vi "WPI_ERRMotorControlCANJaguarFirmware.vi"(0 "error code":i32, 7 "Device Number":u8, 9 "minimum firmware version":u32, 11 "current firmware version":u32) -> (8 "error out":errorcluster)   [LabVIEW 2017]
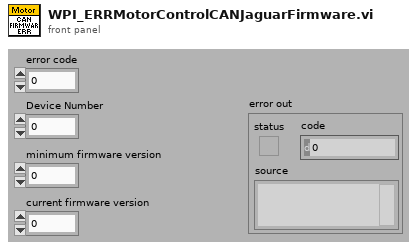
[diagram p1: front panel]
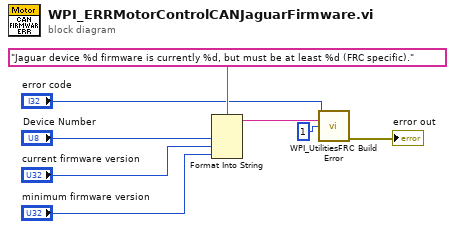
[diagram p0: block diagram]
diagram:
  n1 = Format Into String(format string="Jaguar device %d firmware is currently %d, but must be at least %d (FRC specific).", "Device Number", "current firmware version", "minimum firmware version") -> (resulting string=w4:string)  [unwired: 2 in, 1 out]
  n2 = call <vilib>:"WPI_UtilitiesFRC Build Error.vi"("error code"="error code", "extra error text"=w4, "chain levels to remove (1)"=1) -> ("error out"=→"error out":errorcluster)  [unwired: 2 in, 10 out]
